vi "Start motor controller.vi"(7 "node-ID":u8, 8 "error in (no error)":errorcluster, 11 "interface object in":refnum<k20>) -> (0 "error out":errorcluster, 2 "SDO object out":refnum<k20>, 3 "interface object out":refnum<k20>)   [LabVIEW 2016]
uses:
  <vilib>/CANopenLib/CANOPEN.llb/CANopen SDO Create.vi
  Set mode of operation.vi
  Set control mode.vi
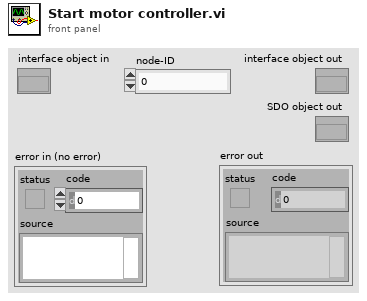
[diagram p1: front panel]
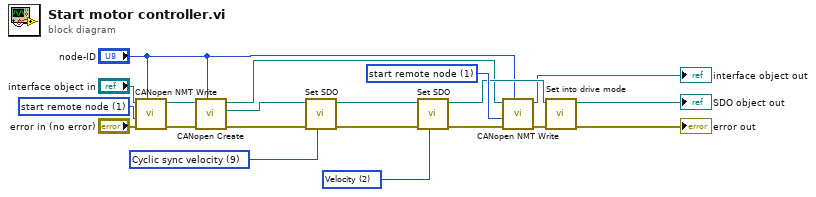
[diagram p0: block diagram]
diagram:
  w13 = u16 1 items=["start remote node"=1, "stop remote node"=2, "enter pre-operational"=128, "reset node"=129, "reset communication"=130] ("command")
  w18 = u8 2 items=["Velocity"=2, "Torque"=1] ("Control Mode")
  w19 = i8 9 items=["Induction VF – testing purposes only"=-5, "Aligning rotor position"=-4, "Current stepper – testing purposes only "=-3, "Voltage stepper – testing purposes only"=-2, "Voltage constant angle – testing purposes only"=-1, "No mode"=0, "Cyclic sync position"=8, "Cyclic sync velocity"=9, "Cyclic sync torque"=10] ("Mode of operation")
  w20 = u16 1 items=["start remote node"=1, "stop remote node"=2, "enter pre-operational"=128, "reset node"=129, "reset communication"=130] ("command")
  n1 = call <vilib>:"CANopen NMT Write.vi"("node-ID (0)"="node-ID", "error in (no error)"="error in (no error)", "command"=w20, "interface object in"="interface object in") -> ("error out"=w4:errorcluster, "interface object out"=w9:refnum<k20>)  [unwired: 6 in]
  n2 = call-poly <vilib>:"CANopen Create.vi"("node-ID"="node-ID", "error in (no error)"=w4, "interface object in"=w9) -> ("error out"=w17:errorcluster, "SDO object out"=w16:refnum<k20>, "interface object out"=w8:refnum<k20>)  [unwired: 6 in]
  n3 = call-poly "Set SDO.vi"("Mode of operation"=w19, "error in (no error)"=w17, "SDO object in"=w16) -> ("error out"=w14:errorcluster, "SDO object out"=w15:refnum<k20>)  [unwired: 6 in, 1 out]
  n4 = call-poly "Set SDO.vi"("Control Mode"=w18, "error in (no error)"=w14, "SDO object in"=w15) -> ("error out"=w12:errorcluster, "SDO object out"=w10:refnum<k20>)  [unwired: 6 in, 1 out]
  n5 = call <vilib>:"CANopen NMT Write.vi"("node-ID (0)"="node-ID", "error in (no error)"=w12, "command"=w13, "interface object in"=w8) -> ("error out"=w11:errorcluster, "interface object out"=→"interface object out":refnum<k20>)  [unwired: 6 in]
  n6 = call "Set into drive mode.vi"("error in (no error)"=w11, "SDO object in"=w10) -> ("error out"=→"error out":errorcluster, "SDO object out"=→"SDO object out":refnum<k20>)  [unwired: 8 in]
